vi "Tabela_dinamica.vi"() -> ()   [LabVIEW 2013]
panel:
  in  "ContadorEstado":u8=1 min=1
  in  "ContadorBase":u8=1 min=1
  in  "SortearEstado":bool
  in  "SortearBase":bool
  out "Bases e Estados":string[][](table)=[["", "1", "2", "3", "4", "5", "6", "7", "8", "9", "10", "11", "12", "13", "14", "15", "16", "17", "18", "19", "20"], ["Base", "", "", "", "", "", "", "", "", "", "", "", "", "", "", "", "", "", "", "", ""], ["Estado", "", "", "", "", "", "", "", "", "", "", "", "", "", "", "", "", "", "", "", ""]] caption="Sorteio das bases e valores medidos"
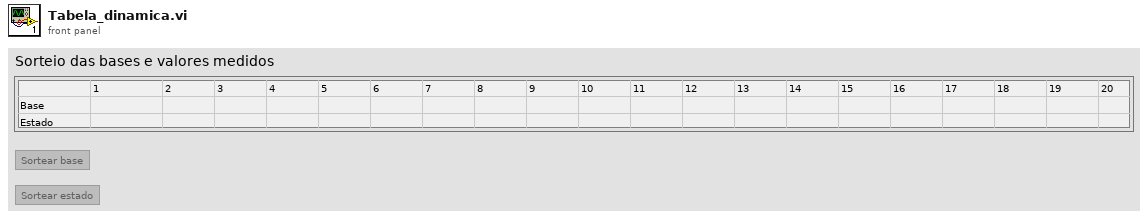
[diagram p1: front panel]
types:
  T1 = enum8{"Enabled", "Disabled", "Disabled and Grayed Out"}
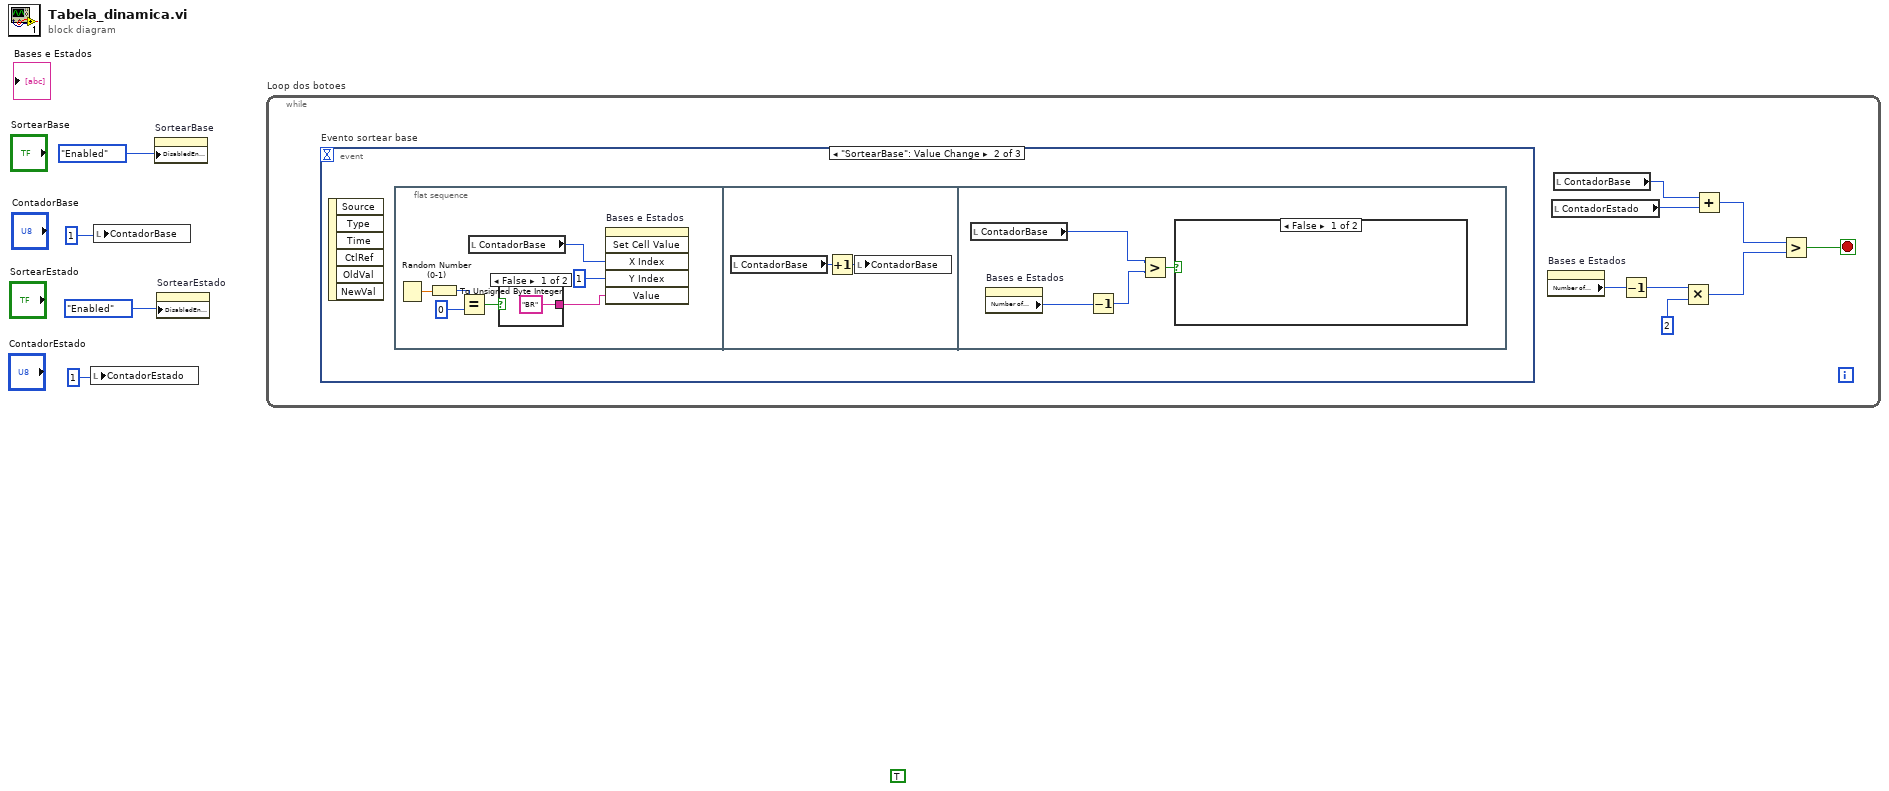
[diagram p0: block diagram]
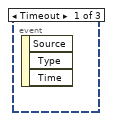
[diagram p2: hidden frame]
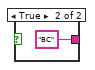
[diagram p3: hidden frame]
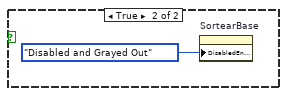
[diagram p4: hidden frame]
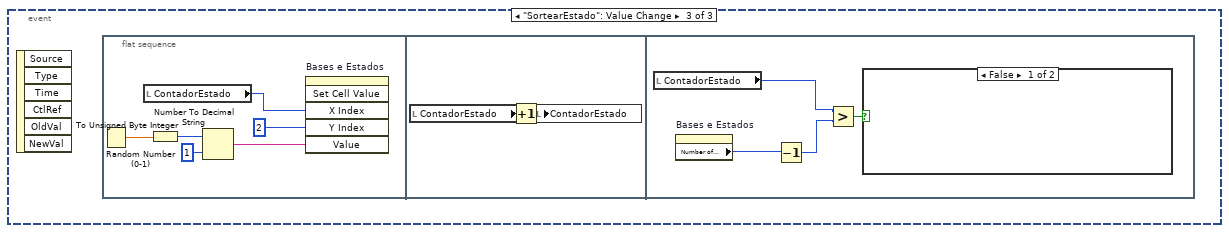
[diagram p5: hidden frame]
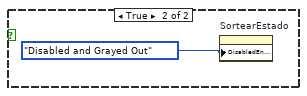
[diagram p6: hidden frame]
diagram:
  (unwired) TRUE
  n1 = local write "ContadorEstado"(u8 1 ("ContadorEstado")) -> ()
  n2 = local write "ContadorBase"(u8 1 ("ContadorBase")) -> ()
  n3 = property on="SortearBase" class="Bool"("DisabledEnum"=T1."Enabled" ("Disabled")) -> ()  [unwired: 2 in, 2 out]
  n4 = property on="SortearEstado" class="Bool"("DisabledEnum"=T1."Enabled" ("Disabled")) -> ()  [unwired: 2 in, 2 out]
  n5 = while "Loop dos botoes" {
    stop <- w7 stop-if-true
    n6 = event "Evento sortear base" shown="[1] \"SortearBase\": Value Change" {
      selector: _ -> [_ _ _]
      dyn-events: _ -> [_ _ _]
      timeout: _ -> [_ _ _]
      event Timeout {
        n7 = event-data() -> ()  [unwired: 1 in, 3 out]
      }
      event "SortearBase": Value Change {
        n8 = event-data() -> ()  [unwired: 1 in, 6 out]
        n9 = flat-sequence {
          frame #0 {
            n10 = Random Number (0-1)() -> (number: 0 to 1=w19:dbl)
            n11 = To Unsigned Byte Integer(number=w19) -> (unsigned 8bit integer=w16:u8)
            n12 = Equal?(x=w16, y=u8 0) -> (x = y?=w15:bool)
            n13 = local read "ContadorBase"() -> (w17:u8)
            n14 = case shown="False" w15 {
              tunnel: ["BR" "BC"] -> w13
              frame False {
              }
              frame True {
              }
            }
            n15 = invoke on="Bases e Estados" class="Tbl (strict)" method="Set Cell Value"("X Index"=w17, "Y Index"=1, "Value"=w13) -> ()  [unwired: 3 in, 6 out]
          }
          frame #1 {
            n16 = local read "ContadorBase"() -> (w23:u8)
            n17 = Increment(x=w23) -> (x+1=w22:u8)
            n18 = local write "ContadorBase"(w22) -> ()
          }
          frame #2 {
            n19 = local read "ContadorBase"() -> (w26:u8)
            n20 = property on="Bases e Estados" class="Tbl (strict)"() -> ("Number of Columns"=w27:u32)  [unwired: 2 in, 2 out]
            n21 = Decrement(x=w27) -> (x-1=w25:u32)
            n22 = Greater?(x=w26, y=w25) -> (0:w24:bool)
            n23 = case shown="False" w24 {
              frame False {
              }
              frame True {
                n24 = property on="SortearBase" class="Bool"("DisabledEnum"=T1."Disabled and Grayed Out" ("Disabled")) -> ()  [unwired: 2 in, 2 out]
              }
            }
          }
        }
      }
      event "SortearEstado": Value Change {
        n25 = event-data() -> ()  [unwired: 1 in, 6 out]
        n26 = flat-sequence {
          frame #0 {
            n27 = Random Number (0-1)() -> (number: 0 to 1=w34:dbl)
            n28 = local read "ContadorEstado"() -> (w29:u8)
            n29 = To Unsigned Byte Integer(number=w34) -> (unsigned 8bit integer=w33:u8)
            n30 = Number To Decimal String(number=w33, width (-)=i16 1) -> (decimal integer string=w31:string)
            n31 = invoke on="Bases e Estados" class="Tbl (strict)" method="Set Cell Value"("X Index"=w29, "Y Index"=2, "Value"=w31) -> ()  [unwired: 3 in, 6 out]
          }
          frame #1 {
            n32 = local read "ContadorEstado"() -> (w36:u8)
            n33 = Increment(x=w36) -> (x+1=w35:u8)
            n34 = local write "ContadorEstado"(w35) -> ()
          }
          frame #2 {
            n35 = local read "ContadorEstado"() -> (w40:u8)
            n36 = property on="Bases e Estados" class="Tbl (strict)"() -> ("Number of Columns"=w37:u32)  [unwired: 2 in, 2 out]
            n37 = Decrement(x=w37) -> (x-1=w39:u32)
            n38 = Greater?(x=w40, y=w39) -> (0:w38:bool)
            n39 = case shown="False" w38 {
              frame False {
              }
              frame True {
                n40 = property on="SortearEstado" class="Bool"("DisabledEnum"=T1."Disabled and Grayed Out" ("Disabled")) -> ()  [unwired: 2 in, 2 out]
              }
            }
          }
        }
      }
    }
    n41 = property on="Bases e Estados" class="Tbl (strict)"() -> ("Number of Columns"=w9:u32)  [unwired: 2 in, 2 out]
    n42 = local read "ContadorEstado"() -> (w11:u8)
    n43 = local read "ContadorBase"() -> (w12:u8)
    n44 = Decrement(x=w9) -> (x-1=w8:u32)
    n45 = Multiply(x=w8, y=u32 2) -> (x*y=w5:u32)
    n46 = Add(x=w12, y=w11) -> (x+y=w6:u8)
    n47 = Greater?(x=w6, y=w5) -> (0:w7:bool)
  }
